vi "TDMS_loading_speeds_test.vi"() -> ()   [LabVIEW 2016]
panel:
  in  "create index file? (T)":bool
  out "Loaded data":T1
  in  "Data samples to load":i64=100
  out "Time to load data only, ms":u32
  out "Full load time, ms":u32
  in  "file path":path=path "C:/Users/Dmitriy/Documents/MHC_Tracker/Track_2018-10-05-18-23-21/SavedTrack-2018-10-05-18-23-21.tdms"
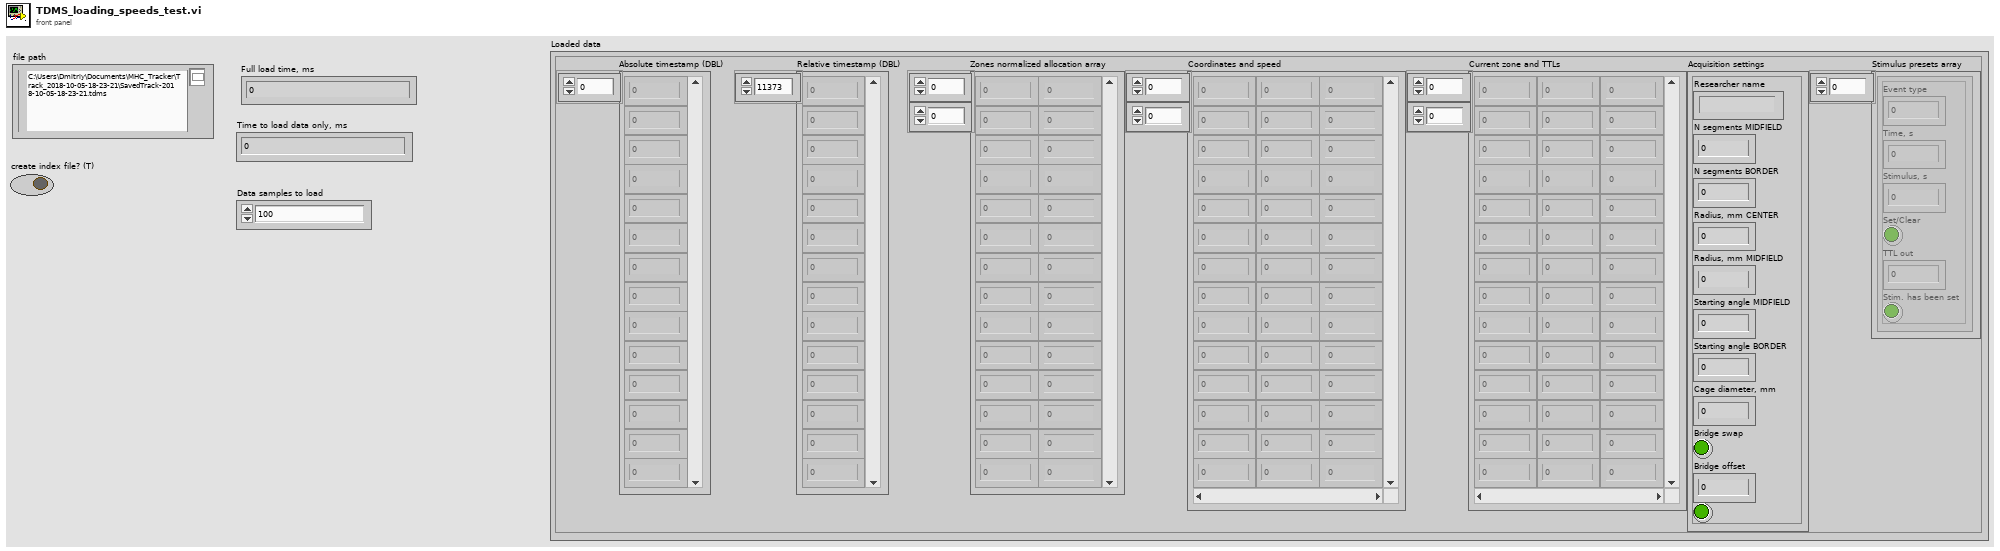
[diagram p1: front panel]
types:
  T1 = cluster{"Absolute timestamp (DBL)":dbl[], "Relative timestamp (DBL)":dbl[], "Zones normalized allocation array":dbl[][], "Coordinates and speed":dbl[][], "Current zone and TTLs":u8[][], "Acquisition settings":cluster{"Researcher name":string, "N segments MIDFIELD":u8, "N segments BORDER":u8, "Radius, mm CENTER":u16, "Radius, mm MIDFIELD":u16, "Starting angle MIDFIELD":i16, "Starting angle BORDER":i16, "Cage diameter, mm":u16, "Bridge swap":bool, "Bridge offset":sgl, "Boolean":bool}, "Stimulus presets array":cluster{"Event type":u16, "Time, s":sgl, "Stimulus, s":sgl, "Set/Clear":bool, "TTL out":u16, "Stim. has been set":bool}[]}
  T2 = cluster{"Data acquisition status":refnum<notifier>, "Play/Pause status":refnum<notifier>, "Complete stop":refnum<notifier>, "Temp file ready for processing":refnum<notifier>, "Has been recorded":refnum<notifier>, "Recording now":refnum<notifier>, "Path to the latest complete temp file":refnum<notifier>, "Final CSV saved":refnum<notifier>, "Data loaded":refnum<notifier>}
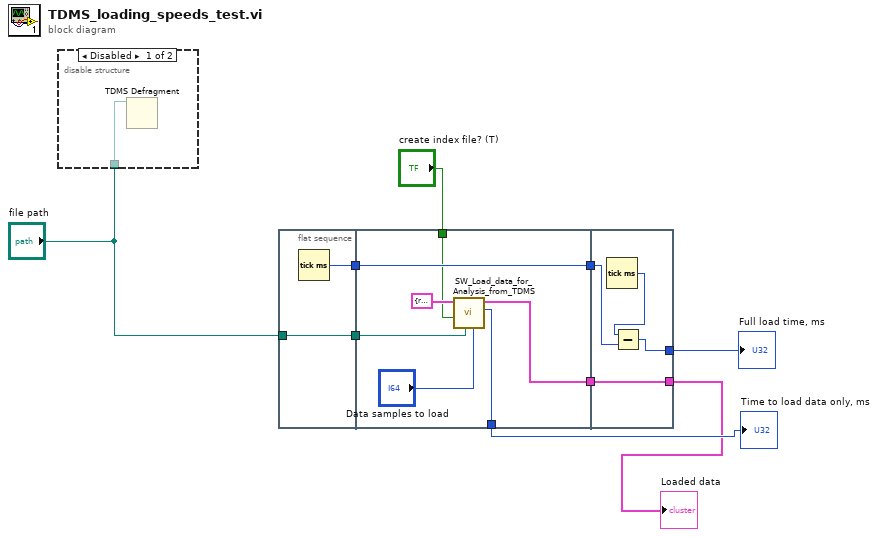
[diagram p0: block diagram]
diagram:
  n1 = disable-structure shown="Disabled" {
    disable-tunnel: "file path" -> [w10 _]
    frame Disabled {
      n2 = TDMS Defragment(7:w10) -> ()  [unwired: 1 in, 1 out]
    }
    frame Enabled {
    }
  }
  n3 = flat-sequence {
    tunnel: "file path" -> [w12]
    tunnel: [w12] -> w8
    tunnel: [w11] -> w7
    tunnel: w8 -> [w19]
    tunnel: [w16] -> w6
    tunnel: w7 -> [w16]
    tunnel: [w15] -> w3
    tunnel: "create index file? (T)" -> [w14]
    tunnel: [w13] -> w5
    tunnel: w6 -> [w22]
    tunnel: [w21] -> w4
    tunnel: w5 -> [w20]
    tunnel: [w20] -> w1
    frame #0 {
      n4 = Tick Count (ms)() -> (millisecond timer value=w11:u32)
    }
    frame #1 {
      n5 = call "SW_Load_data_for_Analysis_from_TDMS.vi"("create index file? (T)"=w14, "Data samples to load"="Data samples to load", "Path to TDMS file"=w19, "Data flow controls"=T2 {"Data acquisition status"=refnum, "Play/Pause status"=refnum, "Complete stop"=refnum, "Temp file ready for processing"=refnum, "Has been recorded"=refnum, "Recording now"=refnum, "Path to the latest complete temp file"=refnum, "Final CSV saved"=refnum, "Data loaded"=refnum}) -> ("Time to load, ms"=w15:u32, "Loaded data"=w13:T1)  [unwired: 3 in, 3 out]
    }
    frame #2 {
      n6 = Tick Count (ms)() -> (millisecond timer value=w23:u32)
      n7 = Subtract(x=w23, y=w22) -> (x-y=w21:u32)
    }
  }
  "Full load time, ms" <- w4
  "Time to load data only, ms" <- w3
  "Loaded data" <- w1
